vi "OEE_SCREEN_1_recolor_pace.vi"(1 "pace_field_reference":refnum<vi>, 2 "pace_value":string) -> ()   [LabVIEW 2019]
uses:
  FGV/SQL_raw_data/FGV_OEE_SQL_raw_data.ctl
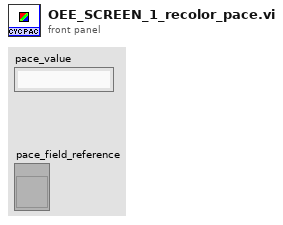
[diagram p1: front panel]
types:
  T1 = typedef "FGV_OEE_SQL_raw_data.ctl" = enum16{"initialize", "set_reference_name", "set_timestamp", "set_OK_NOK_count", "set_config_info", "set_pace", "set_availability", "set_hourly_ok_count", "set_targets", "get_all_info"}
  T2 = typedef "OEE_SQL_raw_data.ctl" = cluster{"reference_name":string, "data_timestamp":timestamp, "OK_NOK_count":string[][], "config_info":string[], "pace":string[][], "availability":string[], "hourly_ok_count":string[][], "shift_number":i8, "shift_start":i8, "shift_end":i8, "TAKT":u16, "FTTH_target":u16, "BOTTLENECK_station":string, "targets_hourly":u16[], "target_shift":u16}
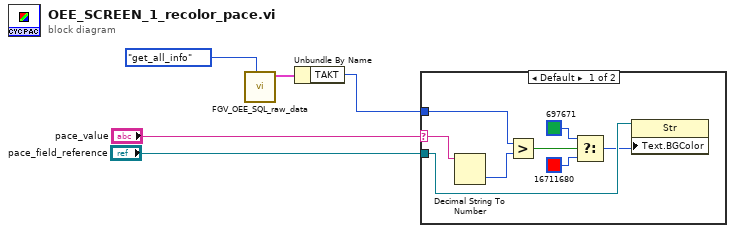
[diagram p0: block diagram]
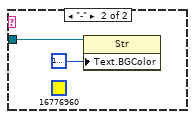
[diagram p2: hidden frame]
diagram:
  n1 = call "FGV_OEE_SQL_raw_data.vi"("options"=FGV_OEE_SQL_raw_data."get_all_info") -> ("SQL_raw_data_out"=w5:T2)  [unwired: 9 in, 1 out]
  n2 = Unbundle By Name(w5) -> ("TAKT"=w1:u16)
  n3 = case shown="Default" "pace_value" {
    selector: "pace_value" -> [w13 _]
    tunnel: "pace_field_reference" -> [w10 w14]
    tunnel: w1 -> [w11 _]
    frame Default {
      n4 = Decimal String To Number(string=w13) -> (number=w12:i32)  [unwired: 2 in, 1 out]
      n5 = Greater?(x=w11, y=w12) -> (0:w7:bool)
      n6 = Select(t=u32 697671, s=w7, f=u32 16711680) -> (s? t:f=w6:u32)
      n7 = property class="Str"(reference=w10, "Text.BGColor"=w6) -> ()  [unwired: 1 in, 2 out]
    }
    frame "-" {
      (unwired) u32 16776960
      n8 = property class="Str"(reference=w14, "Text.BGColor"=u32 16777228) -> ()  [unwired: 1 in, 2 out]
    }
  }
